vi "Set Rx Async.vi"(8 "error in":errorcluster, 10 "rx async?":bool, 11 "Ballard ARINC 429 custom device in":T1 format="%.0x") -> (0 "error out":errorcluster, 3 "Ballard ARINC 429 custom device out":T1 format="%.0x")   [LabVIEW 2020, in "Ballard ARINC 429 Scripting.lvlib"]
doc: "Writes the <b>description</b> field for the input <b>Ballard ARINC 429 custom device</b>."
uses:
  Ballard ARINC 429 Scripting.lvlib
  <vilib>/NI VeriStand/Custom Device API/Custom Device Item Ref.ctl
  Constants.vi
  <vilib>/NI VeriStand/Custom Device API/Set Item Property (Boolean).vi
  <vilib>/NI VeriStand/Custom Device API/Custom Device API.lvlib
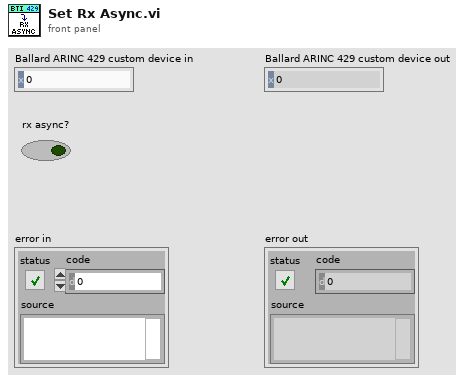
[diagram p1: front panel]
types:
  T1 = typedef "Custom Device API.lvlib/Custom Device Item Ref.ctl" = u64
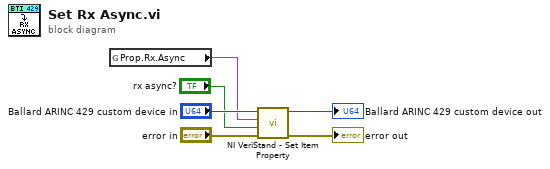
[diagram p0: block diagram]
diagram:
  n1 = global read "Constants.vi" "Prop.Rx.Async"() -> (w1:string)
  n2 = call-poly <vilib>:"NI VeriStand - Set Item Property.vi"("error in (no error)"="error in", "Value"="rx async?", "Property Name"=w1, "Item Ref in"="Ballard ARINC 429 custom device in") -> ("error out"=→"error out":errorcluster, "Item Ref out"=→"Ballard ARINC 429 custom device out":T1)  [unwired: 5 in, 1 out]
